vi "Initialize.vi"(8 "error in":errorcluster, 11 "Ballard ARINC-429 Rx Execution Unit in":refnum<class "Ballard ARINC-429 Rx Execution Unit.lvclass">) -> (0 "error out":errorcluster, 3 "Ballard ARINC-429 Rx Execution Unit out":refnum<class "Ballard ARINC-429 Rx Execution Unit.lvclass">)   [LabVIEW 2020, in "Ballard ARINC 429 Engine.lvlib" / "Implementation.lvlib" / "Ballard ARINC-429 Rx Execution Unit.lvclass"]
uses:
  Ballard ARINC-429 Rx Execution Unit.lvclass
  Ballard ARINC-429 Rx Execution Unit.lvclass/Ballard ARINC-429 Rx Execution Unit.ctl
  Custom Device/Custom Device.lvlib
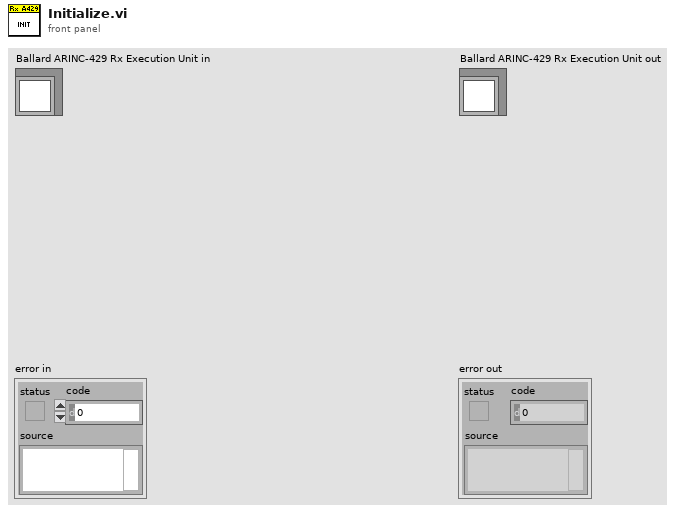
[diagram p1: front panel]
types:
  T1 = typedef "RT Hardware Channel Settings.ctl" = cluster{"channel #":u16, "channel handle":u64, "labels settings for RT":T2[]}
  T2 = typedef "RT Label Settings.ctl" = cluster{"Name":string, "xmlName":string, "label":T3, "transfer period":u32, "SDI_Enabled":bool, "SDI":u8, "parameter driver data":T4, "transfer type":T10, "has timestamp?":bool, "Label Disable/Trigger Channel Reference":T9, "Message Handle":u64, "Initialized?":bool, "Word Initial Raw Value":u32, "Label Timestamp Channel Data Reference":T8}
  T3 = typedef "Label.ctl" = u8
  T4 = typedef "RT Parameters.ctl" = cluster{"parameter definitions":T5[], "Rx block data refs":T7[], "Rx values":dbl[], "Tx parameter refs":T9[]}
  T5 = typedef "Parameter Definition.ctl" = cluster{"start index":i32, "size":i32, "encoding":T6, "signed":bool, "scale multiplier":dbl, "scale offset":dbl}
  T6 = typedef "Encoding and Decoding.lvlib/Encoding.ctl" = enum16{"BNR", "BCD", "Discrete"}
  T7 = typedef "Custom Device API.lvlib/Block Data Reference.ctl" = cluster{"Data Reference":T8, "Offset":u64, "Length":u64}
  T8 = typedef "Custom Device API.lvlib/Data Reference.ctl" = i32
  T9 = typedef "Custom Device API.lvlib/Custom Device Item Ref.ctl" = u64
  T10 = typedef "Transfer Type.ctl" = enum16{"Scheduled", "Acyclic", "Block", "Strobe"}
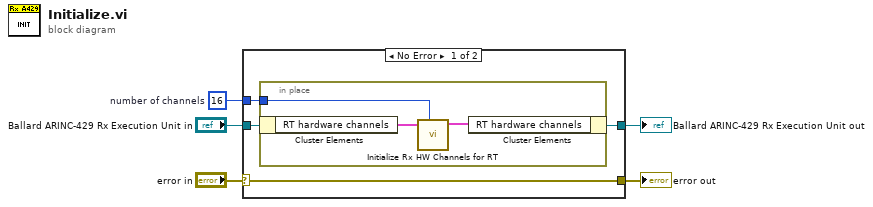
[diagram p0: block diagram]
diagram:
  w3 = 16  # number of channels
  n1 = case shown="No Error" "error in" {
    selector: "error in" -> [w6 w14]
    tunnel: "Ballard ARINC-429 Rx Execution Unit in" -> [w9 w13]
    tunnel: [w8 w13] -> w4
    tunnel: w3 -> [w7 _]
    tunnel: [w6 w14] -> w2
    frame No Error {
      n2 = in-place {
        in-place-border: w7 -> [w10]
        n3 = in-place-cluster #1(w9) -> ("RT hardware channels"=w12:T1[])
        n4 = call "Initialize Rx HW Channels for RT.vi"("number of channels"=w10, "Rx Channels In"=w12) -> ("Rx Channels Out"=w11:T1[])  [unwired: 7 in]
        n5 = in-place-cluster #1("RT hardware channels"=w11) -> (w8:refnum<class "Ballard ARINC-429 Rx Execution Unit.lvclass">)
      }
    }
    frame Error {
    }
  }
  "error out" <- w2
  "Ballard ARINC-429 Rx Execution Unit out" <- w4
